vi "solution2.vi"() -> ()   [LabVIEW 2015]
panel:
  out "?":dbl
  in  "BREADTH":dbl
  in  "lENGTH":dbl
  in  "WIDTH":dbl
  in  "stop":bool
  # "Surface area of cuboid"
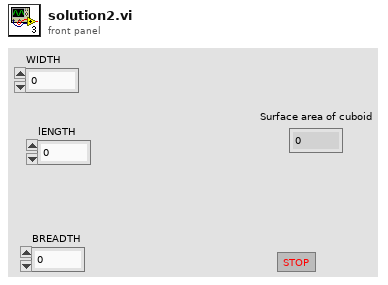
[diagram p1: front panel]
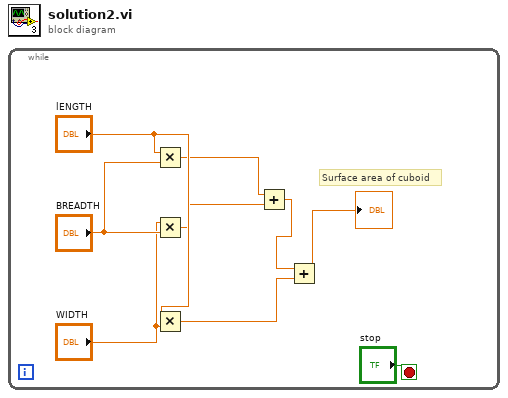
[diagram p0: block diagram]
diagram:
  n1 = while {
    stop <- "stop" stop-if-true
    # "Surface area of cuboid"
    n2 = Multiply(x="lENGTH", y="BREADTH") -> (x*y=w5:dbl)
    n3 = Multiply(x="WIDTH", y="BREADTH") -> (x*y=w4:dbl)
    n4 = Multiply(x="lENGTH", y="WIDTH") -> (x*y=w3:dbl)
    n5 = Add(x=w5, y=w4) -> (x+y=w2:dbl)
    n6 = Add(x=w2, y=w3) -> (x+y=→"?":dbl)
  }
